vi "Find Global Min on Surface_Func.vi"(9 "output selector":T1, 10 "data":variant, 11 "X":dbl[](array[numeric])) -> (0 "error out":errorcluster, 1 "Inequality Constraints":dbl[](array[numeric]), 2 "Equality Constraints":dbl[](array[numeric]), 3 "Objective Functions":dbl[](array[numeric]))   [LabVIEW 2023]
doc: "Finds the global minimum on a surface using the formula illustrated on the block diagram."
uses:
  <vilib>/gmath/NumericalOptimization/cno_output select.ctl
  <vilib>/gmath/NI_Gmath.lvlib
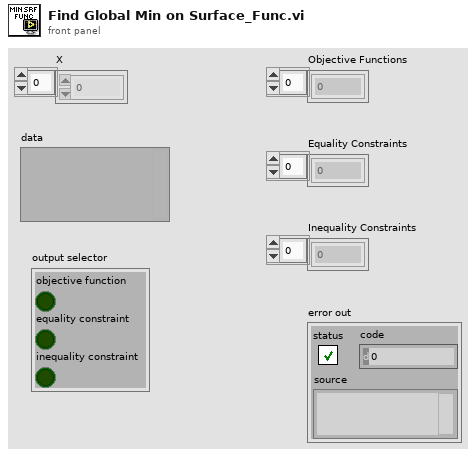
[diagram p1: front panel]
types:
  T1 = typedef "NI_Gmath.lvlib/cno_output select.ctl" = cluster{"objective function":bool, "equality constraint":bool, "inequality constraint":bool}
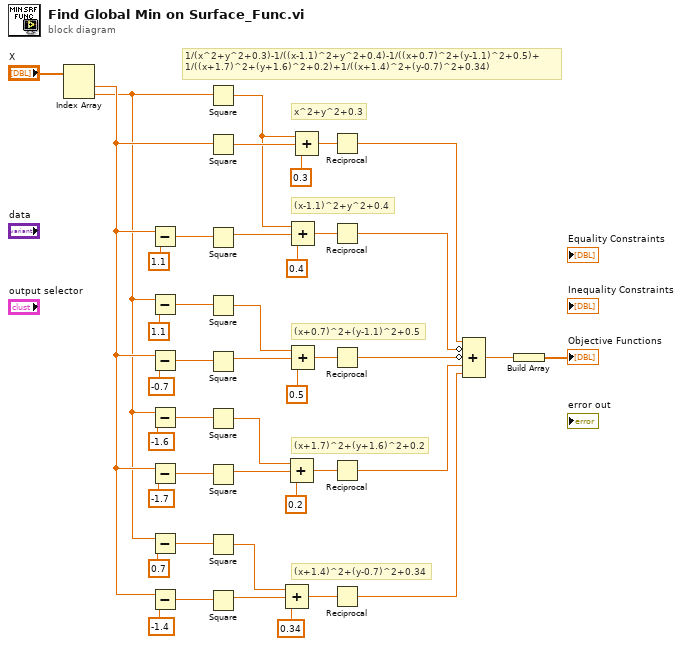
[diagram p0: block diagram]
diagram:
  # "1/(x^2+y^2+0.3)-1/((x-1.1)^2+y^2+0.4)-1/((x+0.7)^2+(y-1.1)^2+0.5)+\n1/((x+1.7)^2+(y+1.6)^2+0.2)+1/((x+1.4)^2+(y-0.7)^2+0.34)"
  # "(x+1.4)^2+(y-0.7)^2+0.34"
  # "(x+1.7)^2+(y+1.6)^2+0.2"
  # "(x+0.7)^2+(y-1.1)^2+0.5"
  # "(x-1.1)^2+y^2+0.4"
  # "x^2+y^2+0.3"
  n1 = Index Array(array="X") -> (element #1=w4:dbl, element #2=w3:dbl)  [unwired: 2 in]
  n2 = Subtract(x=w4, y=1.1) -> (x-y=w41:dbl)
  n3 = Subtract(x=w3, y=1.1) -> (x-y=w26:dbl)
  n4 = Subtract(x=w4, y=-0.7) -> (x-y=w28:dbl)
  n5 = Subtract(x=w3, y=-1.6) -> (x-y=w22:dbl)
  n6 = Subtract(x=w4, y=-1.7) -> (x-y=w20:dbl)
  n7 = Subtract(x=w3, y=0.7) -> (x-y=w8:dbl)
  n8 = Subtract(x=w4, y=-1.4) -> (x-y=w10:dbl)
  n9 = Square(x=w3) -> (x^2=w33:dbl)
  n10 = Square(x=w4) -> (x^2=w37:dbl)
  n11 = Square(x=w41) -> (x^2=w38:dbl)
  n12 = Square(x=w26) -> (x^2=w25:dbl)
  n13 = Square(x=w28) -> (x^2=w31:dbl)
  n14 = Square(x=w22) -> (x^2=w23:dbl)
  n15 = Square(x=w20) -> (x^2=w17:dbl)
  n16 = Square(x=w8) -> (x^2=w7:dbl)
  n17 = Square(x=w10) -> (x^2=w13:dbl)
  n18 = Compound Arithmetic op=ADD(w7, w13, 0.34) -> (w14:dbl)
  n19 = Compound Arithmetic op=ADD(w23, w17, 0.2) -> (w16:dbl)
  n20 = Compound Arithmetic op=ADD(w33, w38, 0.4) -> (w36:dbl)
  n21 = Compound Arithmetic op=ADD(w25, w31, 0.5) -> (w32:dbl)
  n22 = Compound Arithmetic op=ADD(w33, w37, 0.3) -> (w42:dbl)
  n23 = Reciprocal(x=w42) -> (1/x=w35:dbl)
  n24 = Reciprocal(x=w36) -> (1/x=w34:dbl)
  n25 = Reciprocal(x=w32) -> (1/x=w24:dbl)
  n26 = Reciprocal(x=w16) -> (1/x=w15:dbl)
  n27 = Reciprocal(x=w14) -> (1/x=w6:dbl)
  n28 = Compound Arithmetic op=ADD(w35, invert w34, invert w24, w15, w6) -> (w2:dbl)
  n29 = Build Array(w2) -> (→"Objective Functions":dbl[])
